vi "NF LI56xx u_switch by data type.vi"(0 "Num":u8, 2 "data format":enum16{"ASCii", "REAL", "INTeger"}(ring), 4 "input string":string) -> (15 "query measurement data":dbl[](array[numeric]))   [LabVIEW 2019]
doc: "read data by appropriate data format"
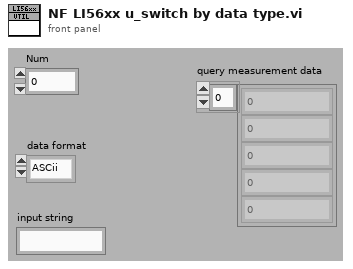
[diagram p1: front panel]
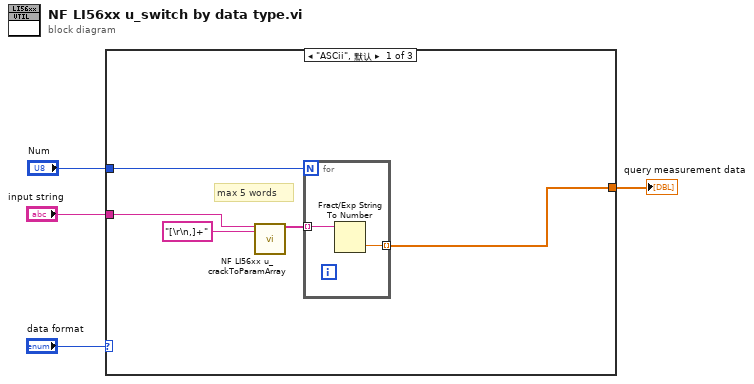
[diagram p0: block diagram]
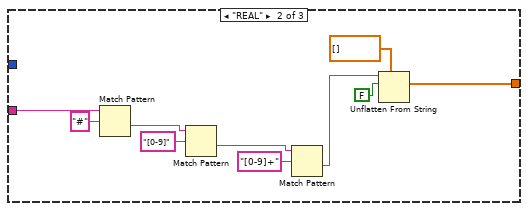
[diagram p2: hidden frame]
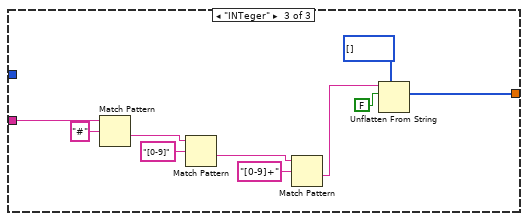
[diagram p3: hidden frame]
diagram:
  n1 = case shown="\"ASCii\", 默认" "data format" {
    tunnel: "Num" -> [w7 _ _]
    tunnel: "input string" -> [w6 w15 w27]
    tunnel: [w5 w16 w22] -> w1
    frame "ASCii", Default {
      # "max 5 words"
      n2 = call "NF LI56xx u_crackToParamArray.vi"("answerParam"=w6, "delimiter"="[\r\n,]+") -> ("paramArray"=w8:string[])  [unwired: 17 in]
      n3 = for {
        N: w7 -> [_]
        tunnel: [w11] -> w5 mode=indexing
        tunnel: w8 -> [w10] mode=indexing
        n4 = Fract/Exp String To Number(string=w10) -> (number=w11:dbl)  [unwired: 3 in, 1 out]
      }
    }
    frame "REAL" {
      n5 = Match Pattern(string=w15, regular expression="#" ("³K\\»")) -> (after substring=w14:string)  [unwired: 1 in, 3 out]
      n6 = Match Pattern(string=w14, regular expression="[0-9]" ("³K\\»")) -> (after substring=w13:string)  [unwired: 1 in, 3 out]
      n7 = Match Pattern(string=w13, regular expression="[0-9]+" ("³K\\»")) -> (after substring=w12:string)  [unwired: 1 in, 3 out]
      n8 = Unflatten From String(type=dbl[] [], binary string=w12, data includes array or string size? (T)=FALSE ("データは配列または文字列サイズを含む?（T）")) -> (value=w16:dbl[])  [unwired: 2 in, 2 out]
    }
    frame "INTeger" {
      n9 = Match Pattern(string=w27, regular expression="#" ("³K\\»")) -> (after substring=w26:string)  [unwired: 1 in, 3 out]
      n10 = Match Pattern(string=w26, regular expression="[0-9]" ("³K\\»")) -> (after substring=w25:string)  [unwired: 1 in, 3 out]
      n11 = Match Pattern(string=w25, regular expression="[0-9]+" ("³K\\»")) -> (after substring=w24:string)  [unwired: 1 in, 3 out]
      n12 = Unflatten From String(type=i16[] [], binary string=w24, data includes array or string size? (T)=FALSE ("データは配列または文字列サイズを含む?（T）")) -> (value=w22:i16[])  [unwired: 2 in, 2 out]
    }
  }
  "query measurement data" <- w1
